vi "MoveAndSample.vi"() -> ()   [LabVIEW 2017]
panel:
  out "Numeric":i32
  in  "Distance/Sample":dbl
  in  "Axis#":i16 min=0 max=2 step=1
  in  "Forward/Reverse":bool
  out "5V Indicator":bool
  in  "Total Distance (mm)":dbl
  out "Waveform Graph":dynamicdata(graph)
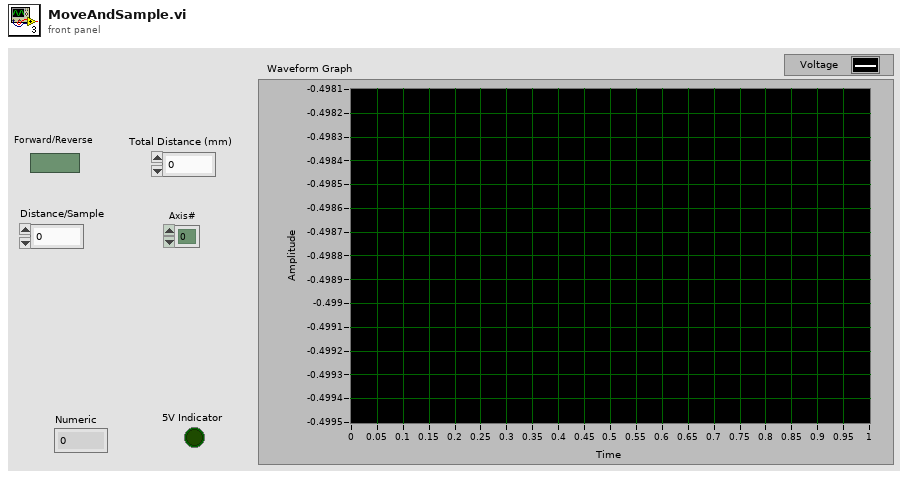
[diagram p1: front panel]
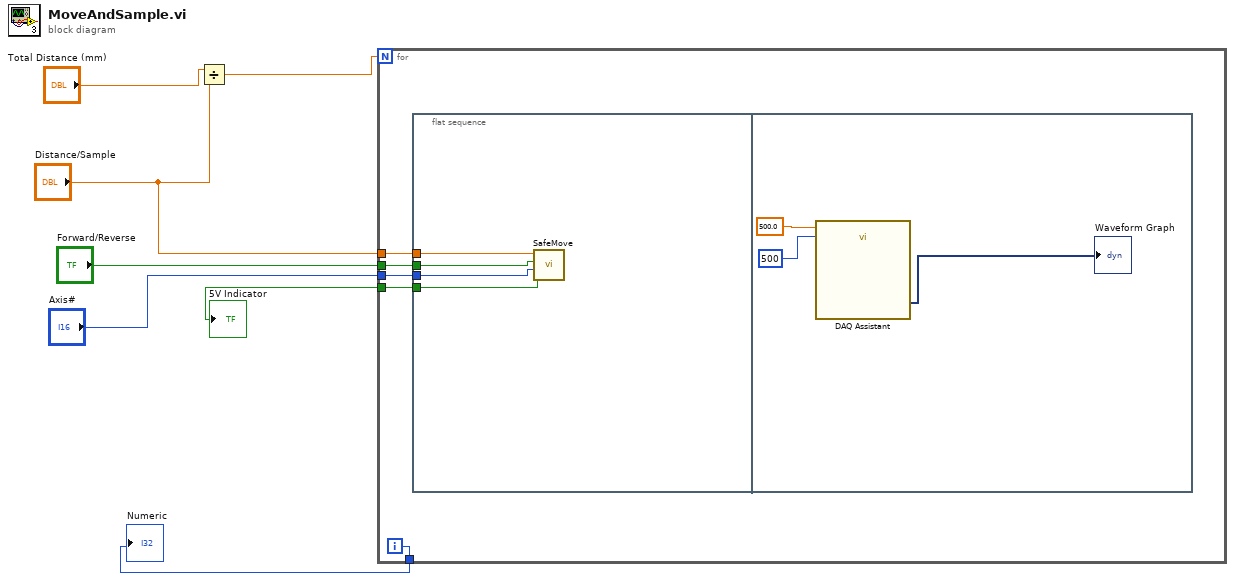
[diagram p0: block diagram]
diagram:
  n1 = Divide(x="Total Distance (mm)", y="Distance/Sample") -> (x/y=w3:dbl)
  n2 = for {
    N: w3 -> [_]
    tunnel: [w12] -> w7
    tunnel: "Forward/Reverse" -> [w11]
    tunnel: "Axis#" -> [w10]
    tunnel: "Distance/Sample" -> [w9]
    tunnel: [w8] -> w1
    i -> [w8]
    n3 = flat-sequence {
      tunnel: [w16] -> w12
      tunnel: w11 -> [w15]
      tunnel: w10 -> [w14]
      tunnel: w9 -> [w13]
      frame #0 {
        n4 = call "SafeMove.vi"("Axis#"=w14, "Forward/Reverse"=w15, "Total Distance (mm)"=w13) -> ("5V Indicator"=w16:bool)  [unwired: 8 in]
      }
      frame #1 {
        n5 = call "DAQ Assistant"("rate"=500.0, "number of samples"=500) -> ("data"=→"Waveform Graph":dynamicdata)  [unwired: 15 in, 2 out]
      }
    }
  }
  "5V Indicator" <- w7
  "Numeric" <- w1
